vi "SetTransparency.vi"(8 "error in (no error)":errorcluster, 10 "Transparency":u8, 11 "FolloWin in":refnum<class "FolloWin.lvclass">) -> (0 "error out":errorcluster, 3 "FolloWin out":refnum<class "FolloWin.lvclass">)   [LabVIEW 2023, in "FolloWin.lvclass"]
doc: "Sets the transparency of the FolloWin window. \nTransparency Values - 0 to 100."
uses:
  FolloWin.lvclass
  FolloWin.lvclass/FolloWin.ctl
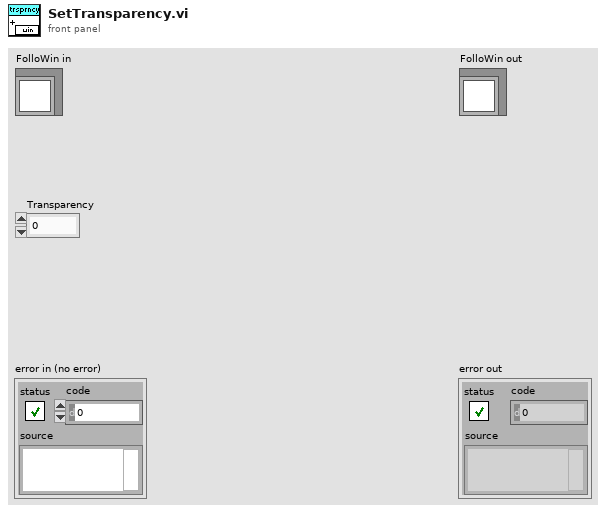
[diagram p1: front panel]
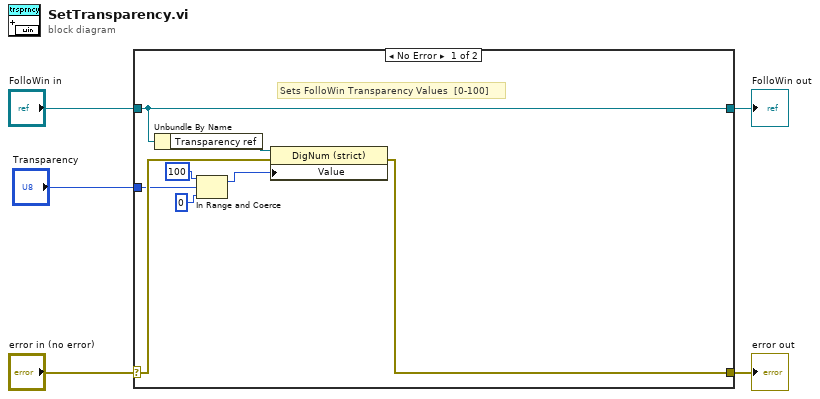
[diagram p0: block diagram]
diagram:
  n1 = case shown="No Error" "error in (no error)" {
    selector: "error in (no error)" -> [w11 w15]
    tunnel: [w10 w15] -> w4
    tunnel: [w13 w14] -> w2
    tunnel: "FolloWin in" -> [w13 w14]
    tunnel: "Transparency" -> [w7 _]
    frame No Error {
      # "Sets FolloWin Transparency Values  [0-100]"
      n2 = Unbundle By Name(w13) -> ("Transparency ref"=w12:refnum<vi>)
      n3 = In Range and Coerce(upper limit=u8 100, x=w7, lower limit=u8 0) -> (coerced(x)=w6:u8)  [unwired: 1 out]
      n4 = property on="Property Node" class="DigNum (strict)"(reference=w12, error in=w11, "Value"=w6) -> (error out=w10:errorcluster)  [unwired: 1 out]
    }
    frame Error {
    }
  }
  "error out" <- w4
  "FolloWin out" <- w2
